vi "Init Device.vi"(8 "error in (no error)":errorcluster, 11 "Device-Thru in":refnum<class "Thru.lvclass">) -> (0 "error out":errorcluster, 3 "Device-Thru out":refnum<class "Thru.lvclass">)   [LabVIEW 2020, in "Thru.lvclass"]
doc: "Init the device com port.\nThis should be called by the child class and the child class is responsible for setting the device as its default state."
uses:
  Thru.lvclass
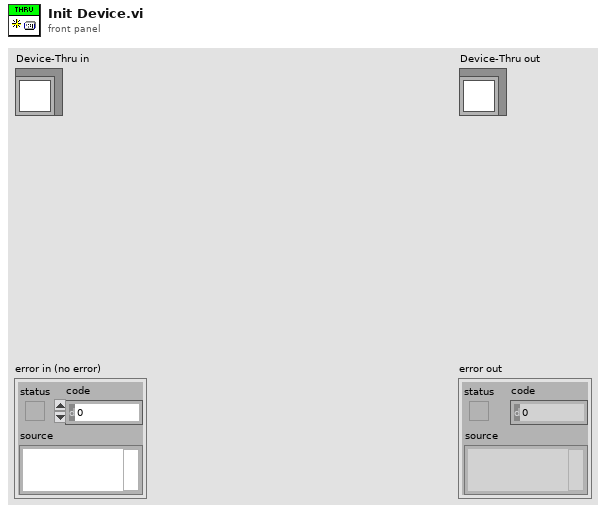
[diagram p1: front panel]
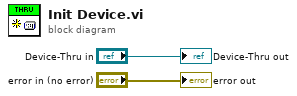
[diagram p0: block diagram]
diagram:
  "error out" <- "error in (no error)"
  "Device-Thru out" <- "Device-Thru in"
